vi "initiate.vi"(0 "reference in":refnum<class "Notification Controller.lvclass">, 5 "error in (no error)":errorcluster) -> (14 "reference out":refnum<class "Notification Controller.lvclass">, 19 "error out":errorcluster)   [LabVIEW 2015, in "Notification Controller.lvclass"]
uses:
  Notification Controller.lvclass
  Devices Controller_llb/Devices Controller.lvclass
  File Controller_llb/File Controller.lvclass
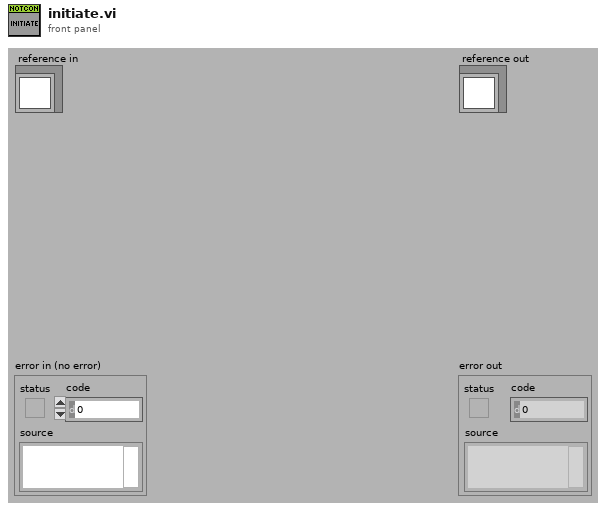
[diagram p1: front panel]
types:
  T1 = typedef "Notification Controller.lvclass/ObjectAttributesRef.ctl" = refnum<data-value>
  T2 = typedef "Notification Controller.lvclass/ObjectAttributes.ctl" = cluster{"MyAttribute":dbl, "items_data":string[][][], "items_notification_refs":refnum<class "itemsNotification.lvclass">[], "notifications_data_items":string[][], "items_nots?":bool, "devices_controller_ref":refnum<class "Devices Controller.lvclass">, "onlineUpdate":timestamp, "notController?":bool, "tracking_notification_ref":refnum<class "trackingNotification.lvclass">, "notifications_data_tracking":string[][], "tracking_parts_data":string[][], "tracking_nots?":bool, "index_tracking_not":i32[], "file_controller_ref":refnum<class "File Controller.lvclass">}
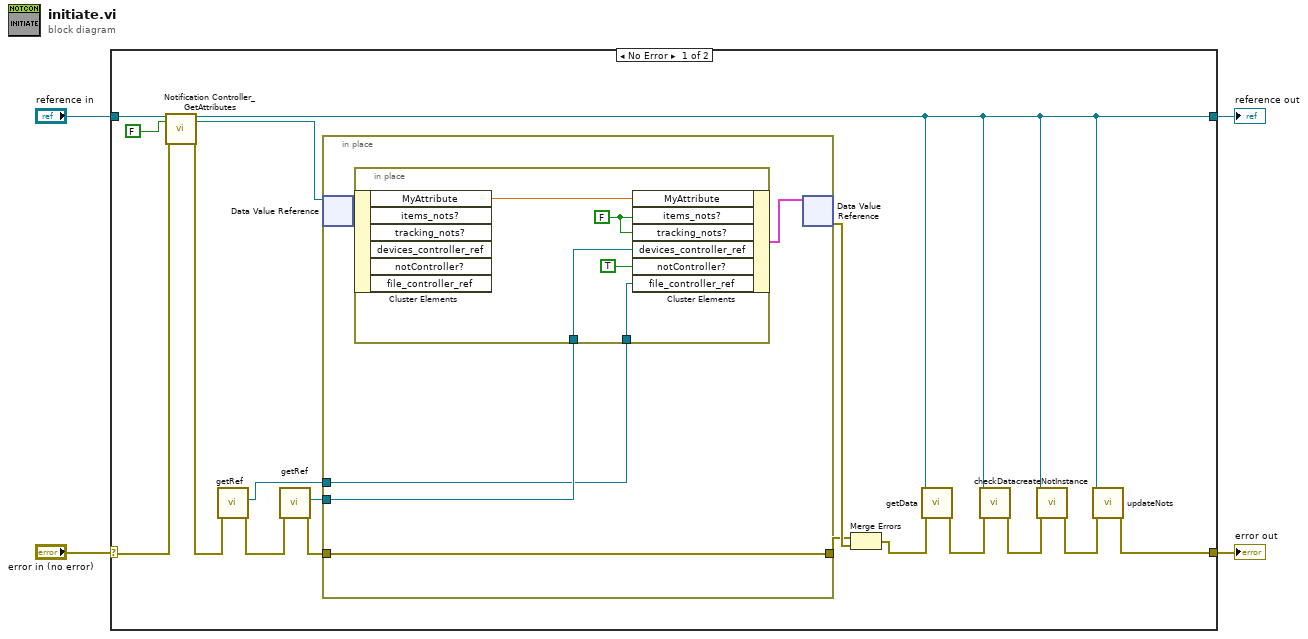
[diagram p0: block diagram]
diagram:
  n1 = case shown="No Error" "error in (no error)" {
    selector: "error in (no error)" -> [w17 w33]
    tunnel: [w12 w33] -> w3
    tunnel: [w11 w32] -> w1
    tunnel: "reference in" -> [w19 w32]
    frame No Error {
      n2 = call "Notification Controller_GetAttributes.vi"("reference in"=w19, "return data? (T)"=FALSE, "error in (no error)"=w17) -> ("reference out"=w11:refnum<class "Notification Controller.lvclass">, "attributes ref"=w16:T1, "error out"=w8:errorcluster)  [unwired: 13 in, 1 out]
      n3 = call "getRef.vi"("error in (no error)"=w8) -> ("error out"=w7:errorcluster, "File Controller_ref"=w6:refnum<class "File Controller.lvclass">)  [unwired: 9 in]
      n4 = call "getRef.vi"("error in (no error)"=w7) -> ("error out"=w10:errorcluster, "device_controller_ref"=w9:refnum<class "Devices Controller.lvclass">)  [unwired: 9 in]
      n5 = in-place {
        in-place-border: w10 -> [w24]
        in-place-border: [w24] -> w20
        in-place-border: w9 -> [w23]
        in-place-border: w6 -> [w22]
        n6 = in-place-dvr #1(w16) -> (w25:T2)  [unwired: 1 out]
        n7 = in-place {
          in-place-border: w23 -> [w29]
          in-place-border: w22 -> [w27]
          w28 = FALSE ("nots?")
          n8 = in-place-cluster #2(w25) -> ("MyAttribute"=w31:dbl)  [unwired: 5 out]
          n9 = in-place-cluster #2("MyAttribute"=w31, "items_nots?"=w28, "tracking_nots?"=w28, "devices_controller_ref"=w29, "notController?"=TRUE, "file_controller_ref"=w27) -> (w26:T2)
        }
        n10 = in-place-dvr #1(w26) -> (w21:errorcluster)  [unwired: 1 out]
      }
      n11 = Merge Errors(w20, w21) -> (w15:errorcluster)
      n12 = call "getData.vi"("error in (no error)"=w15, "reference in"=w11) -> ("error out"=w5:errorcluster)  [unwired: 7 in, 2 out]
      n13 = call "checkData.vi"("error in (no error)"=w5, "reference in"=w11) -> ("error out"=w14:errorcluster)  [unwired: 8 in, 1 out]
      n14 = call "createNotInstance.vi"("error in (no error)"=w14, "reference in"=w11) -> ("error out"=w13:errorcluster)  [unwired: 8 in, 1 out]
      n15 = call "updateNots.vi"("error in (no error)"=w13, "reference in"=w11) -> ("error out"=w12:errorcluster)  [unwired: 8 in, 1 out]
    }
    frame Error {
    }
  }
  "error out" <- w3
  "reference out" <- w1
